vi "Get Configuration File Path.vi"() -> (3 "Configuration File Path":path)   [LabVIEW 2016, in "Assert API Components.lvlib"]
uses:
  Assert API Components/Assert API Components.lvlib
  <vilib>/Utility/sysdir.llb/System Directory Type.ctl
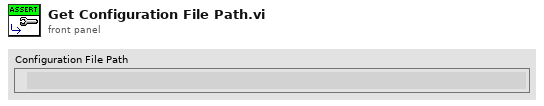
[diagram p1: front panel]
types:
  T1 = typedef "System Directory Type.ctl" = i32
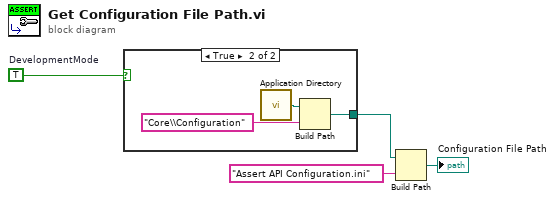
[diagram p0: block diagram]
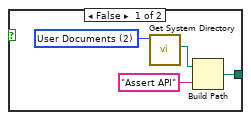
[diagram p2: hidden frame]
diagram:
  w3 = TRUE  # DevelopmentMode
  n1 = case shown="True" w3 {
    tunnel: [w5 w9] -> w4
    frame False {
      w8 = T1 2 items=["User Home"=0, "User Desktop"=1, "User Documents"=2, "User Application Data"=3, "User Preferences"=4, "User Temporary"=5, "Public Documents"=6, "Public Application Data"=7, "Public Preferences"=8, "Public Cache"=13, "System Core Libraries"=9, "System Installed Libraries"=10, "Application Files"=11, "Boot Volume Root"=12] ("system directory type")
      n2 = call <vilib>:"Get System Directory.vi"("system directory type"=w8) -> ("system directory"=w7:path)  [unwired: 10 in]
      n3 = Build Path(base path=w7, name or relative path="Assert API") -> (appended path=w5:path)
    }
    frame True {
      n4 = call <vilib>:"Application Directory.vi"() -> ("Application Directory"=w10:path)
      n5 = Build Path(base path=w10, name or relative path="Core\\Configuration") -> (appended path=w9:path)
    }
  }
  n6 = Build Path(base path=w4, name or relative path="Assert API Configuration.ini") -> (appended path=→"Configuration File Path":path)
